vi "Create Arbitrary Waveform Sequence.vi"(4 "Marker Point":i32[](array[numeric]), 5 "Mark Mode":i32[](array[ring]) items=["Maintain", "Low At Start", "High At Start", "High At Start Go Low"], 6 "Play Control":i32[](array[ring]) items=["Once", "Once Wait Trig", "Repeat", "Repeat Infinitely", "Repeat Till Trig"], 7 "Repeat Count":i32[](array[numeric]), 8 "error in (no error)":errorcluster, 9 "Arbitrary Sequence Waveform Name":string[](array[string]), 10 "Sequence Name (SEQ1)":string="SEQ1", 11 "VISA resource name":refnum<visa-resource-name>) -> (0 "error out":errorcluster, 3 "VISA resource name out":refnum<visa-resource-name>)   [LabVIEW 2020, in "AWG.lvlib" / "Agilent 3352X Series.lvlib"]
doc: "Create an Arbitrary Wavefrom Sequence in volatile memory, use Configure Arbitrary Waveform.vi to load it and change the settings. \n\n<b>Note</b>:\n(1) You can store current loaded seq to non-volatile memory using Store Waveform Data.vi"
uses:
  Agilent 3352X Series.lvlib
panel:
  # "Arbitrary Sequence Data Block"
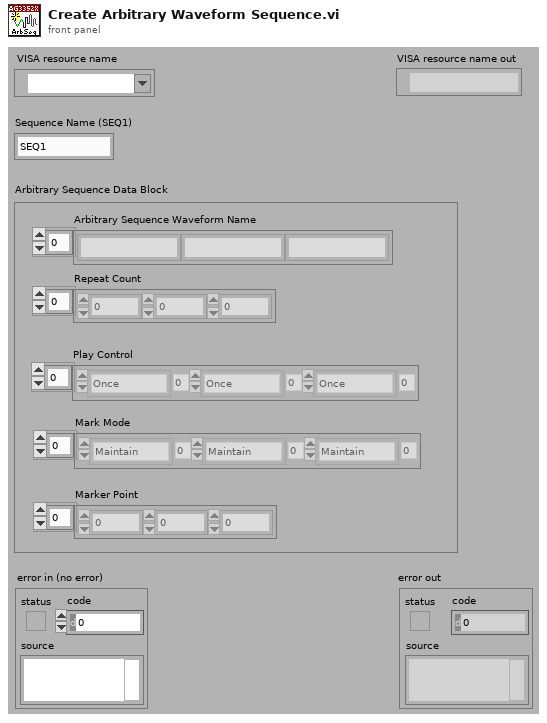
[diagram p1: front panel]
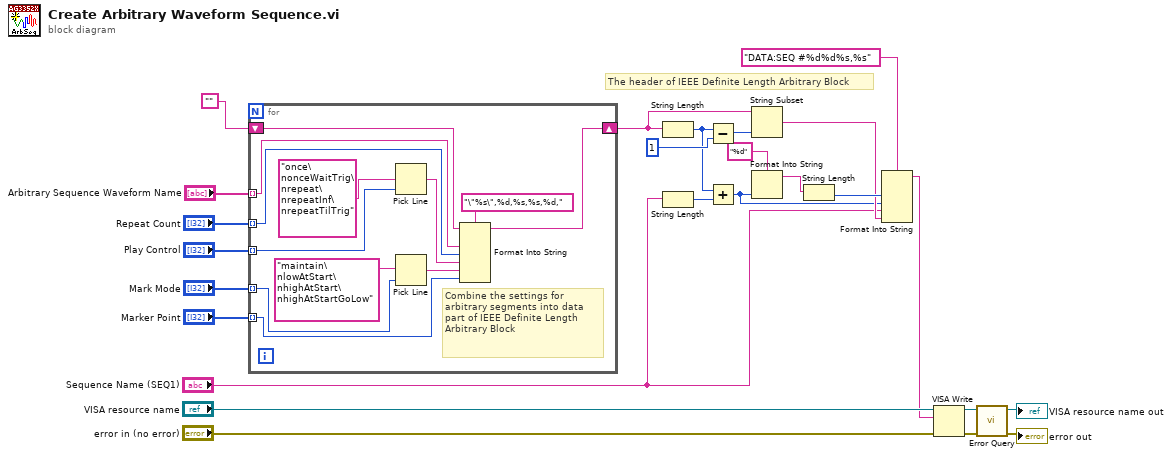
[diagram p0: block diagram]
diagram:
  # "The header of IEEE Definite Length Arbitrary Block"
  n1 = for {
    tunnel: "Arbitrary Sequence Waveform Name" -> [w31] mode=indexing
    tunnel: "Repeat Count" -> [w30] mode=indexing
    tunnel: "Play Control" -> [w36] mode=indexing
    tunnel: "Mark Mode" -> [w35] mode=indexing
    tunnel: "Marker Point" -> [w27] mode=indexing
    shift-right: [w32] -> w14
    shift-left: "" -> [w33]
    # "Combine the settings for arbitrary segments into data part of IEEE Definite Length Arbitrary Block"
    n2 = Pick Line(multi-line string="once\nonceWaitTrig\nrepeat\nrepeatInf\nrepeatTilTrig", line index=w36) -> (output string=w29:string)  [unwired: 1 out]
    n3 = Pick Line(multi-line string="maintain\nlowAtStart\nhighAtStart\nhighAtStartGoLow", line index=w35) -> (output string=w28:string)  [unwired: 1 out]
    n4 = Format Into String(format string="\"%s\",%d,%s,%s,%d,", initial string=w33, w31, w30, w29, w28, w27) -> (resulting string=w32:string)  [unwired: 1 in, 1 out]
  }
  n5 = String Length(string=w14) -> (length=w2:i32)
  n6 = String Length(string="Sequence Name (SEQ1)") -> (length=w3:i32)
  n7 = Subtract(x=w2, y=1) -> (x-y=w10:i32)
  n8 = Add(x=w2, y=w3) -> (x+y=w4:i32)
  n9 = String Subset(string=w14, length (rest)=w10) -> (substring=w7:string)  [unwired: 1 out]
  n10 = Format Into String(format string="%d", w4) -> (resulting string=w9:string)  [unwired: 2 in, 1 out]
  n11 = String Length(string=w9) -> (length=w8:i32)
  n12 = Format Into String(format string="DATA:SEQ #%d%d%s,%s", w8, w4, "Sequence Name (SEQ1)", w7) -> (resulting string=w6:string)  [unwired: 2 in, 1 out]
  n13 = VISA Write(VISA resource name="VISA resource name", write buffer=w6, error in (no error)="error in (no error)") -> (VISA resource name out=w23:refnum<visa-resource-name>, error out=w22:errorcluster)  [unwired: 1 out]
  n14 = call "Error Query.vi"("error in (no error)"=w22, "VISA resource name"=w23) -> ("error out"=→"error out":errorcluster, "VISA resource name out"=→"VISA resource name out":refnum<visa-resource-name>)  [unwired: 8 out]
